vi "DummyNotARefNum.vi"(3 "reference in":refnum<class "G#RealTimeTemplate.lvclass">) -> (0 "not a refnum?":bool, 1 "reference out":refnum<class "G#RealTimeTemplate.lvclass">)   [LabVIEW 2020, in "G#RealTimeTemplate.lvclass"]
doc: "Constructor."
uses:
  <vilib>/addons/_AddQ/G#Templates/G#RealTimeTemplate/G#RealTimeTemplate.lvclass
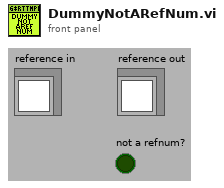
[diagram p1: front panel]
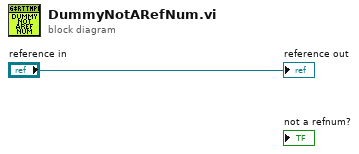
[diagram p0: block diagram]
diagram:
  "reference out" <- "reference in"
